vi "Auto Match.vi"   [LabVIEW 2022 SP3]
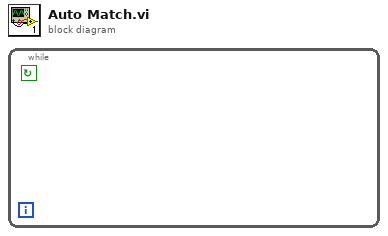
[diagram p0: block diagram]
diagram:
  n1 = while {
    stop <- _ continue-if-true
  }
